vi "AutoRun.vi"(11 "AllControls In":T1) -> ()   [LabVIEW 2017]
uses:
  Ctrls/AllControls.ctl
  Ctrls/Data.ctl
  Ctrls/CSV_Data.ctl
  <vilib>/Utility/miscctls.llb/LVRowAndColumnTypeDef.ctl
  Ctrls/AlarmIndex.ctl
  Ctrls/PathChoose.ctl
  <vilib>/Utility/file.llb/Write Delimited Spreadsheet (string).vi
  <vilib>/regexp/Match Regular Expression.xnode
panel:
  out "Station ID":string
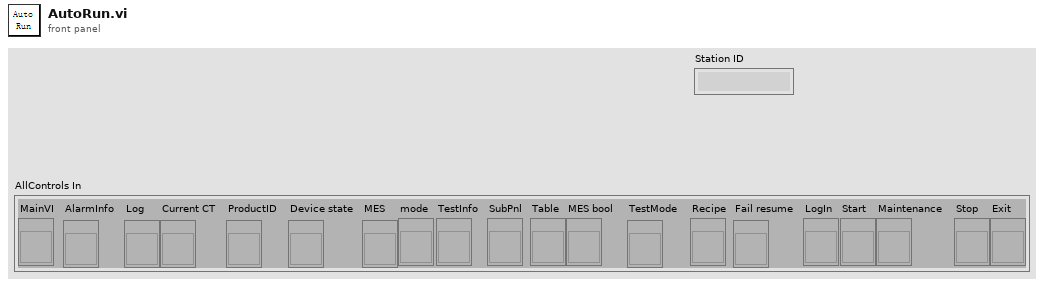
[diagram p1: front panel]
types:
  T1 = typedef "AllControls.ctl" = cluster{"MainVI":refnum<vi>, "AlarmInfo":refnum<vi>, "Log":refnum<vi>, "Current CT":refnum<vi>, "ProductID":refnum<vi>, "Device state":refnum<vi>, "MES":refnum<vi>, "mode":refnum<vi>, "TestInfo":refnum<vi>, "SubPnl":refnum<vi>, "Table":refnum<vi>, "MES bool":refnum<vi>, "TestMode":refnum<vi>, "Recipe":refnum<vi>, "Fail resume":refnum<vi>, "LogIn":refnum<vi>, "Start":refnum<vi>, "Maintenance":refnum<vi>, "Stop":refnum<vi>, "Exit":refnum<vi>}
  T2 = typedef "CSV_Data.ctl" = cluster{"SN":string, "Table":string[][], "Count":cluster{"Total":i32, "OK":i32, "NG":i32, "Yield":dbl}, "Start Time":timestamp, "daemon reference":refnum<k5>, "CT":dbl, "OK/NG":bool, "Station ID":string, "MES DDM SN":string, "MES PCBA SN":string, "Retest":string, "Attachment RFID detection":cluster{"UID":string, "tag content":string}, "SKU":string, "Plate_Diameter":string, "Alarm":string}
  T3 = typedef "Data.ctl" = cluster{"Initialisation":cluster{"DDM_Parameter":dbl[], "DDM_Parameter_status":bool[], "Get_Tester_Parameter":dbl[], "Get_Tester_Parameter_status":bool[], "Cal_Tester_Parameter":dbl[], "Cal_Tester_Parameter_status":bool[], "sw_version_before_status":bool, "sw_version_after_status":bool, "Set_SKU_Config_With_LMT_status":bool, "FCT_timestamp_status":bool, "LMT_Connect_to_UUT_status":bool}, "BEMF_Calibration":cluster{"Read_ambient_temperature":dbl, "Calibration_Vaule":dbl[], "Calibration_Vaule _B":dbl[], "Calibration_Vaule_status":bool[], "Calibration_Vaule_B_status":bool[]}, "ECO":cluster{"DDM_Parameter":dbl[], "DDM_Parameter_status":bool[], "Get_Tester_Parameter":dbl[], "Get_Tester_Parameter_status":bool[], "Cal_Tester_Parameter":dbl[], "Cal_Tester_Parameter_status":bool[], "DDM_Parameter_after_power_tune":dbl[], "Get_Tester_Parameter_after_power_tune":dbl[], "Cal_Tester_Parameter_after_power_tune":dbl[], "Cal_Tester_Parameter_after_power_tune_status":bool[], "Delta_P":dbl}, "BOOST":cluster{"DDM_Parameter":dbl[], "DDM_Parameter_status":bool[], "Get_Tester_Parameter":dbl[], "Get_Tester_Parameter_status":bool[], "Cal_Tester_Parameter":dbl[], "Cal_Tester_Parameter_status":bool[], "DDM_Parameter_after_power_tune":dbl[], "Get_Tester_Parameter_after_power_tune":dbl[], "Cal_Tester_Parameter_after_power_tune":dbl[], "Cal_Tester_Parameter_after_power_tune_status":bool[], "airwatts_am_off":dbl, "AW_Delta_(AM_on_and_off)":dbl, "AW_Delta_(AM_on_and_off)_Status":bool, "Delta_P":dbl}, "MAX":cluster{"Average_Tmag_Data":cluster{"LSI Delta in degC":dbl, "FISF Delta in degc":dbl, "LSI Tmag in degC":dbl, "Fisf Tmag in degC":dbl, "IIR Tmag in degC":dbl}, "DDM_Parameter":dbl[], "DDM_Parameter_status":bool[], "Get_Tester_Parameter":dbl[], "Get_Tester_Parameter_status":bool[], "Cal_Tester_Parameter":dbl[], "BEMF_Finetune":cluster{"eol_bemf_mp_cold_coef_c":dbl, "eol_cold_bemf_fisf_offset":dbl}, "AW_Tune":cluster{"delta_P1":dbl, "delta_P_Setting":dbl}, "DDM_Parameter_after_Airwatts_Tune":dbl[], "Get_Tester_Parameter_after_Airwatts_Tune":dbl[], "Cal_Tester_Parameter_after_Airwatts_Tune":dbl[], "DDM_Parameter_after_Airwatts_Finetune":dbl[], "Get_Tester_Parameter_after_Airwatts_Finetune":dbl[], "Cal_Tester_Parameter_after_Airwatts_Finetune":dbl[], "AW_Finetune":cluster{"delta_P2":dbl, "delta_P_Setting":dbl}, "Delta_Tmag_after_tune":cluster{"LSI Delta in degC":dbl, "FISF Delta in degc":dbl, "LSI Tmag in degC":dbl, "Fisf Tmag in degC":dbl, "IIR Tmag in degC":dbl}, "Hot Bemf in mV":dbl, "DDM_Pressure":dbl, "Delta_Pressure":dbl, " Cold Bemf in mV":dbl, " delta Bemf":dbl, " delta p":dbl, "Delta_Pressure_status":bool, " delta Bemf_status":bool, "LSI Delta in degC_status":bool, "FISF Delta in degc_status":bool, "Max_check_derate_status_status":bool, "Average_All_data":dbl[][], "Average_Tmag_Data_status":bool[], "Average_Tmag_Data_after_tune_status":bool[], "Cal_Tester_Parameter_status":bool[], "Cal_Tester_Parameter_status_after_Airwatts_Tune":bool[], "Cal_Tester_Parameter_status_after_Airwatts_FineTune":bool[]}, "Task_Detect_Calib":cluster{"LL":cluster{"DDM_Parameter":dbl[], "DDM_Parameter_status":bool[], "Get_Tester_Parameter":dbl[], "Get_Tester_Parameter_status":bool[], "Set_task_detect_A":dbl, "Set_task_detect_A_Status":bool}, "HL":cluster{"DDM_Parameter":dbl[], "DDM_Parameter_status":bool[], "Get_Tester_Parameter":dbl[], "Get_Tester_Parameter_status":bool[], "Set_task_detect_B":dbl, "Set_task_detect_B_Status":bool}, "LH":cluster{"DDM_Parameter":dbl[], "DDM_Parameter_status":bool[], "Get_Tester_Parameter":dbl[], "Get_Tester_Parameter_status":bool[], "Set_task_detect_C":dbl, "Set_task_detect_C_Status":bool}, "HH":cluster{"DDM_Parameter":dbl[], "DDM_Parameter_status":bool[], "Get_Tester_Parameter":dbl[], "Get_Tester_Parameter_status":bool[], "Set_task_detect_D":dbl, "Read_and_check_calibration_Status":bool[], "Set_task_detect_D_Status":bool}, "Get_eol_inlet_blockage_E":dbl, "Calib_vaule":cluster{"Get_task_detect_LL":dbl, "Get_task_detect_HL":dbl, "Get_task_detect_LH":dbl, "Get_task_detect_HH":dbl, "eol_inlet_blockage":dbl, "eol_code_bemf_temp":dbl}, "calibrated temp":dbl, "Inlet_Blockage_Calibration":cluster{"DDM_Parameter":dbl[], "DDM_Parameter_status":bool[], "Get_Tester_Parameter":dbl[], "Get_Tester_Parameter_status":bool[]}, "Get_eol_inlet_blockage_E_Status":bool}, "good":cluster{"Write_Product_TS":cluster{"TIMESTAMP":i64, "RIG_ID":i64, "PASSMARK_ID":i64, "PASSMARK_REV":i64}, "Read_Product_TS":cluster{"TIMESTAMP":i64, "RIG_ID":i64, "PASSMARK_ID":i64, "PASSMARK_REV":i64}, "Good_Check_Secuity_Bit_Stauts":bool}}
  T4 = typedef "HD Config.ctl" = cluster{" PC":cluster{"PC Address":u8[], "PC Port":i32}, "FCO":cluster{"COM":refnum<visa-resource-name>, "Baudrate":u32}, "DC Power ":cluster{"COM":refnum<visa-resource-name>, "Baudrate":u32}, "PW3336":cluster{"COM":refnum<visa-resource-name>, "Baudrate":u32}, "Lefoo":cluster{"COM":refnum<visa-resource-name>, "Baudrate":u32}, "AI Model":cluster{"COM":refnum<visa-resource-name>, "Baudrate":u32}, "DIPC":cluster{"COM":refnum<visa-resource-name>}, "RFID":cluster{"IP Address":string, "Port":u16, "Retry":u16}, "Motor":cluster{"COM":refnum<visa-resource-name>, "Baudrate":u32}, "Fail_resume_mode":bool, "GRR":bool}
  T5 = typedef "amc_Message Queue.ctl" = refnum<queue>
  T6 = typedef "TesterInfo.ctl" = cluster{"Station Name":string, "Station Code":string, "ES NO.":string, "Tester ID":string, "PassMark Revision":string, "Rig ID":string, "Deamon_vision":string, "Project Name":string, "FFTesterPath":path, "Enable_User":bool, "Mode":enum16{"682"}, "MES":bool}
  T7 = cluster{"Total":i32, "OK":i32, "NG":i32, "Yield":dbl}
  T8 = typedef "LVRowAndColumnTypeDef.ctl" = cluster{"Row":i32, "Column":i32}
  T9 = enum8{"Enabled", "Disabled", "Disabled and Grayed Out"}
  T10 = typedef "AlarmIndex.ctl" = enum16{"E-Stop", "Safety light grid", "UUT Sealing Cylinder HomePoint", "UUT Sealing Cylinder WorkPoint", "Orifice fixed Cylinder L HomePoint", "Orifice fixed Cylinder L WorkPoint", "Orifice fixed Cylinder R HomePoint", "Orifice fixed Cylinder R WorkPoint", "UUT Cylinder HomePoint", "UUT Cylinder WorkPoint", "Carrier fixed Cylinder L HomePoint", "Carrier fixed Cylinder L WorkPoint", "Carrier fixed Cylinder R HomePoint", "Carrier fixed Cylinder R WorkPoint", "Probe Cylinder HomePoint", "Probe Cylinder WorkPoint", "Motor Error", "Test Error"}
  T11 = typedef "PathChoose.ctl" = enum16{"OperatorLog", "AutoRunLog", "AlmLog", "TestData", "AllTestData", "backup_nvm", "backup_before_flashing"}
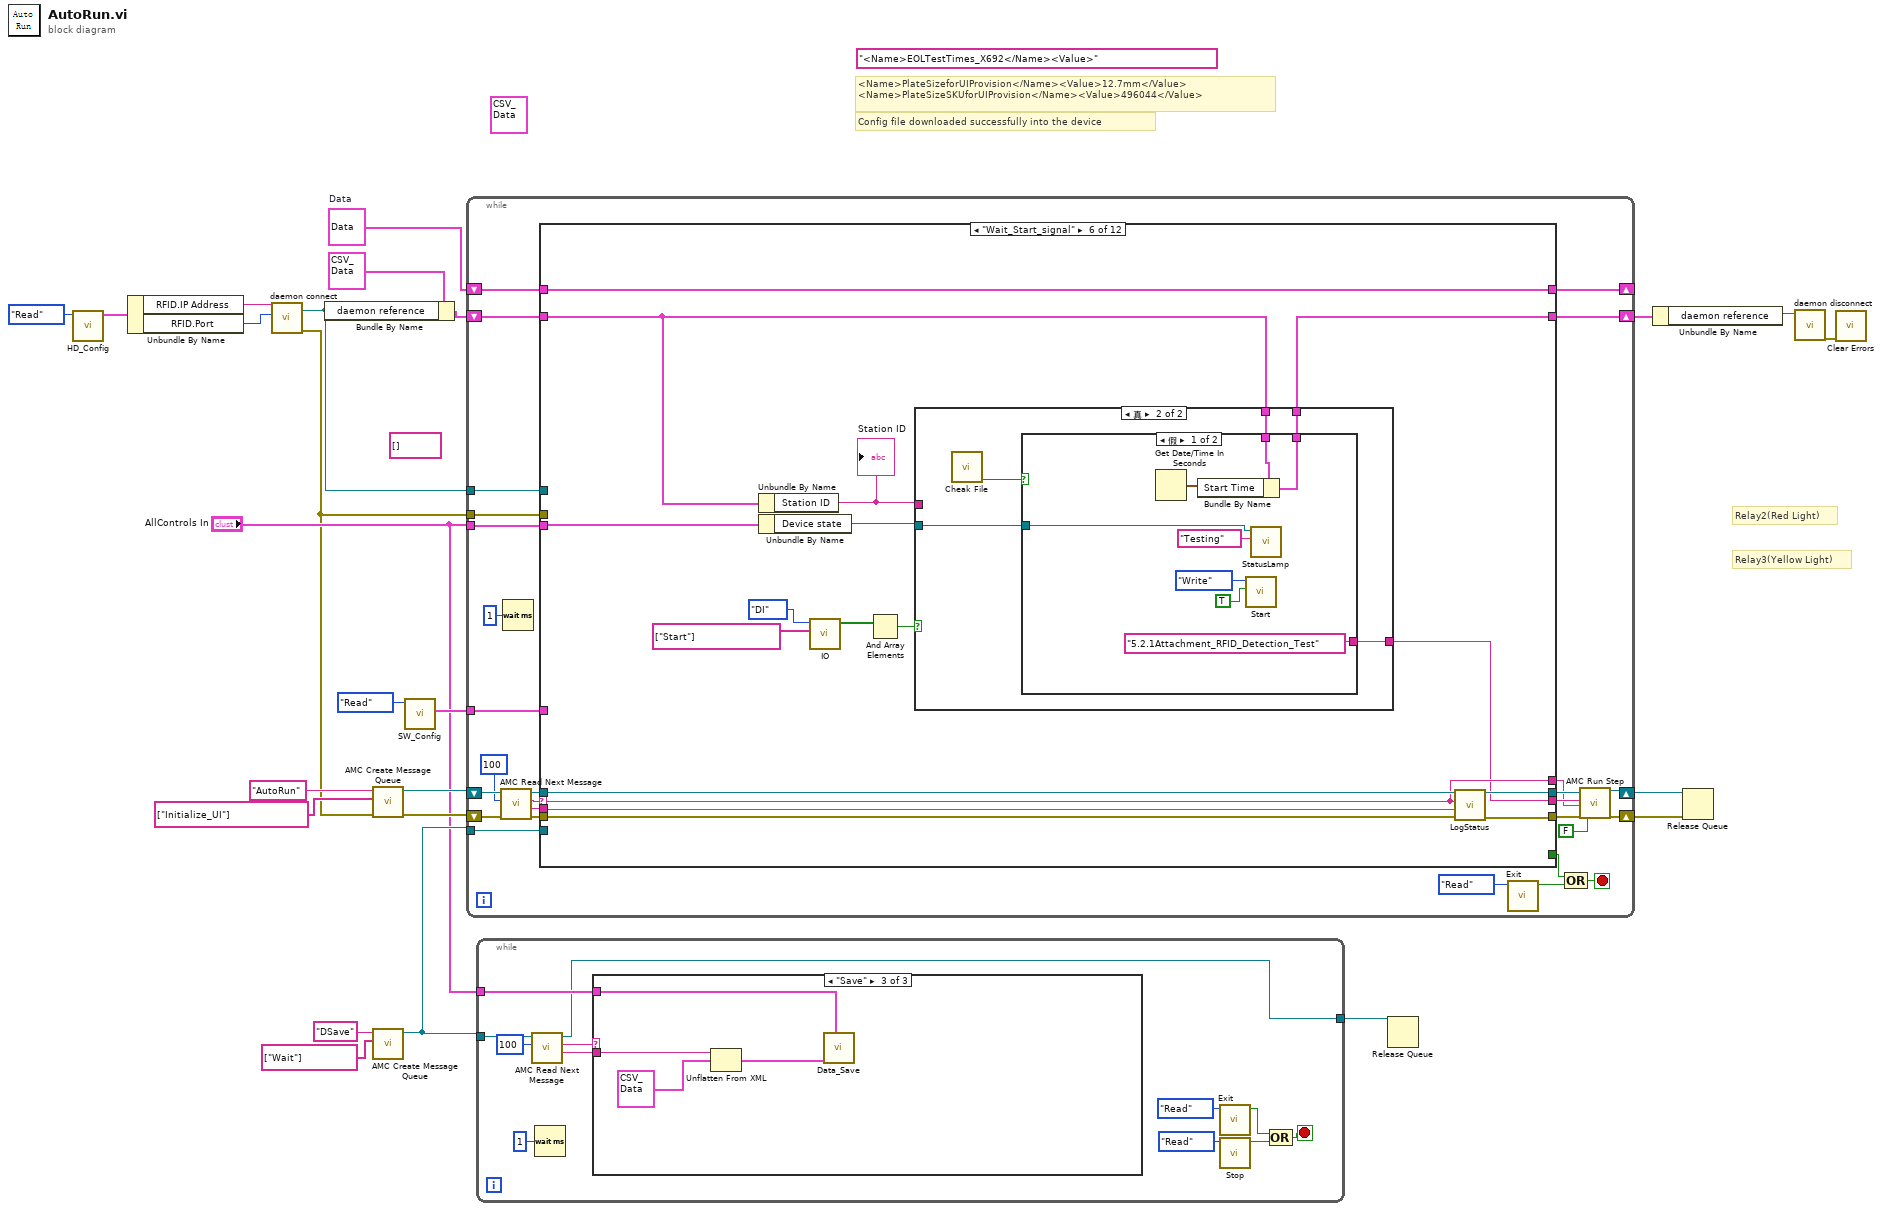
[diagram p0: block diagram]
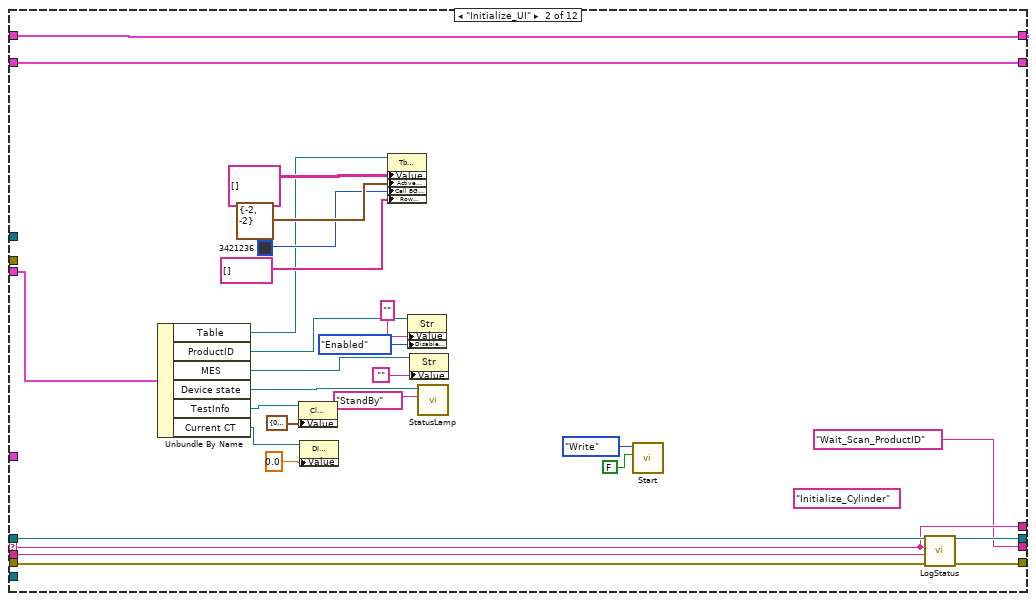
[diagram p5: hidden frame]
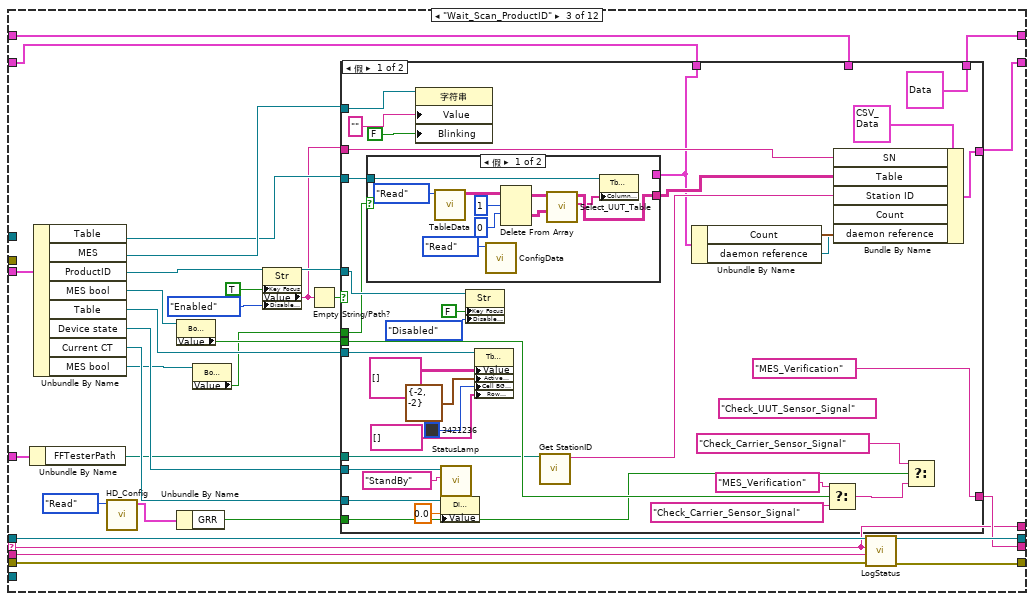
[diagram p6: hidden frame]
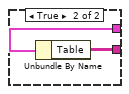
[diagram p7: hidden frame]
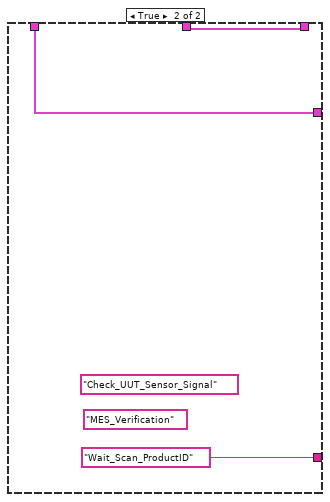
[diagram p8: hidden frame]
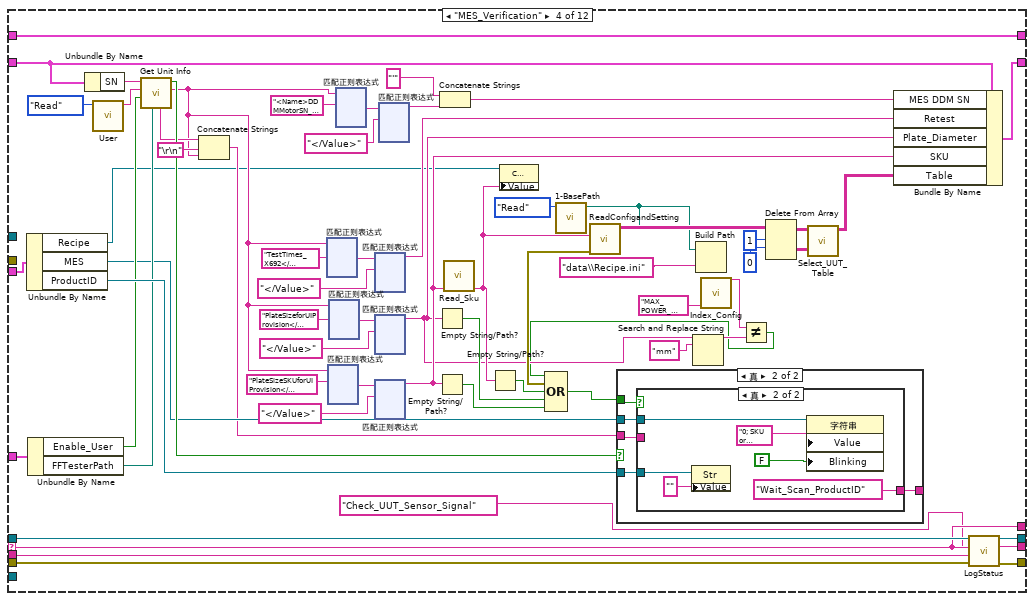
[diagram p9: hidden frame]
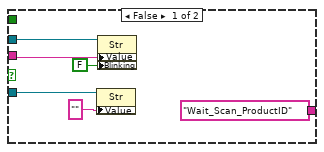
[diagram p10: hidden frame]
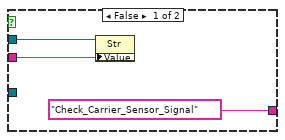
[diagram p11: hidden frame]
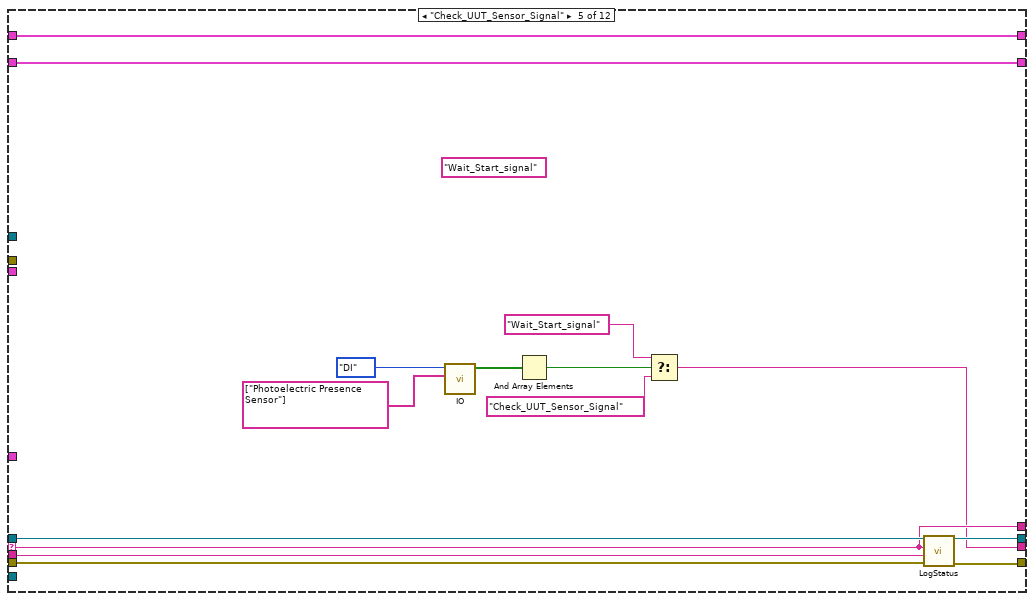
[diagram p12: hidden frame]
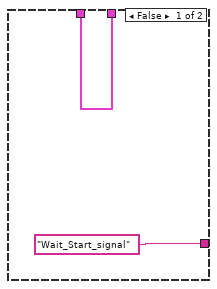
[diagram p13: hidden frame]
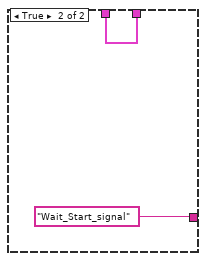
[diagram p14: hidden frame]
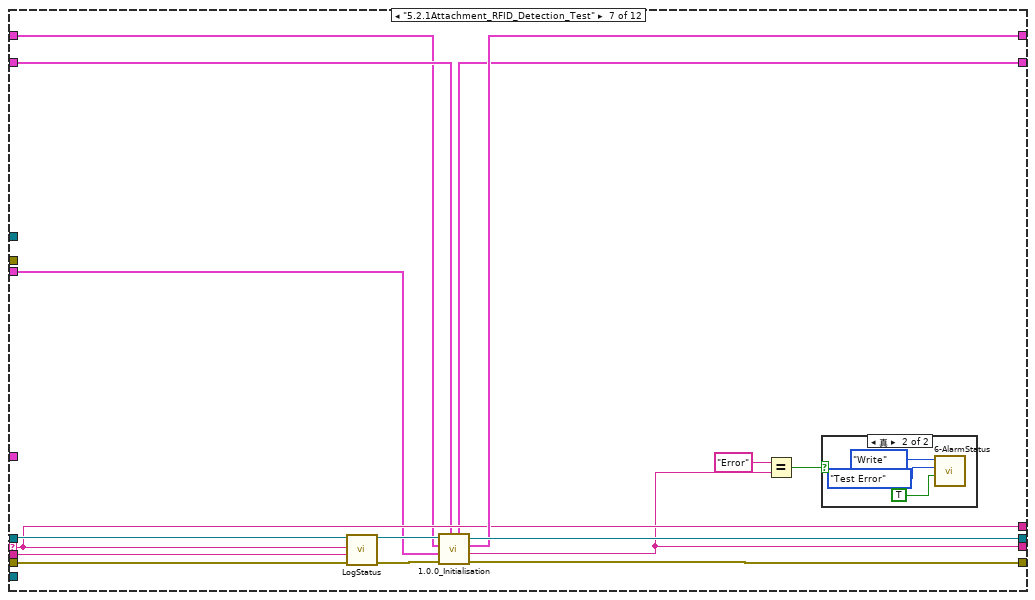
[diagram p15: hidden frame]
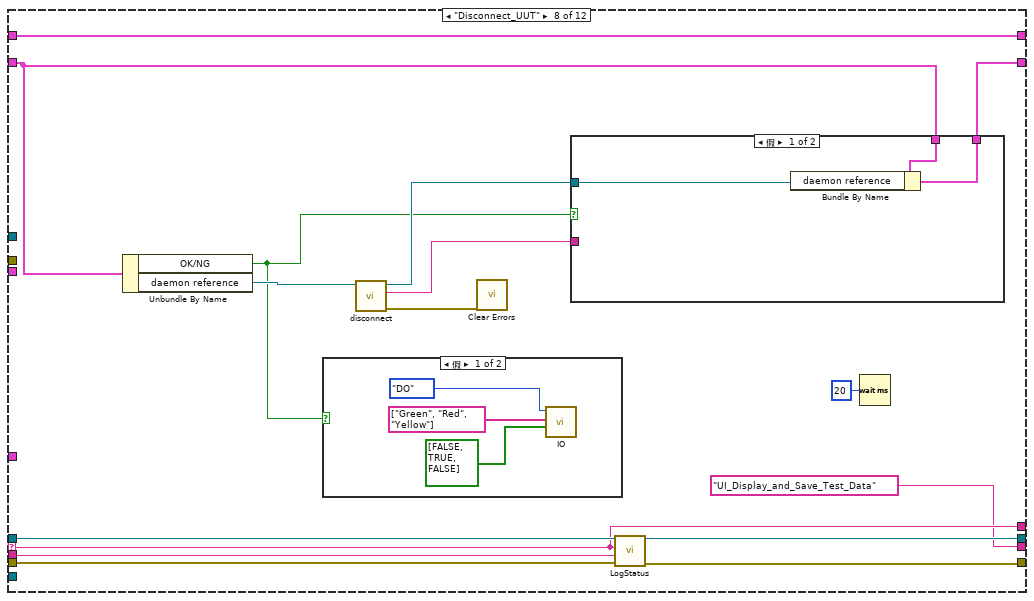
[diagram p17: hidden frame]
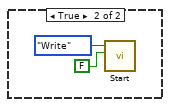
[diagram p18: hidden frame]
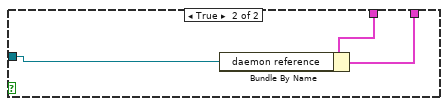
[diagram p19: hidden frame]
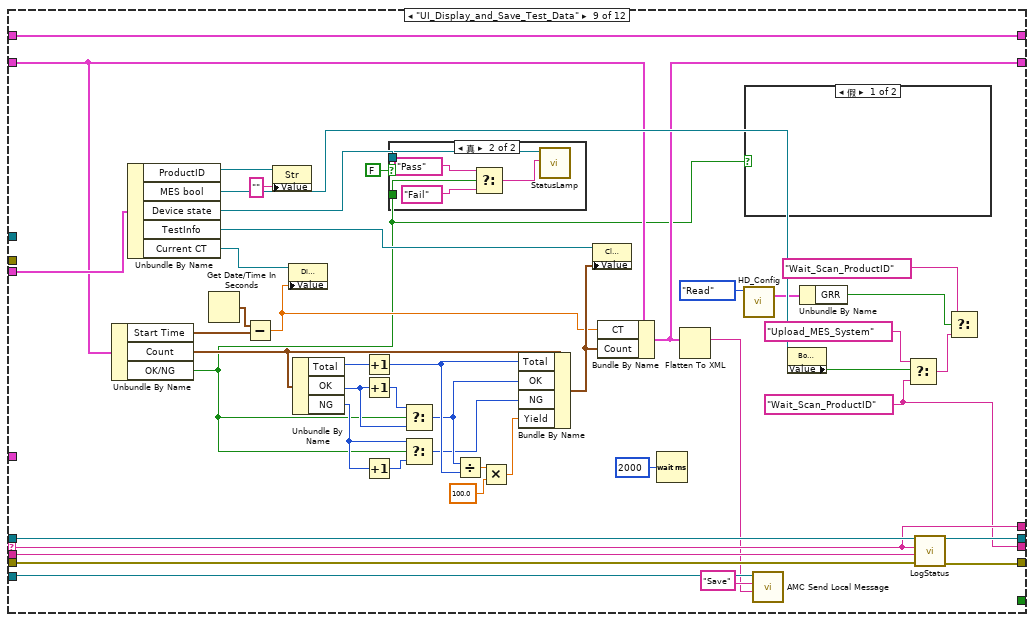
[diagram p20: hidden frame]
diagram:
  (unwired) T2 {"SN"="", "Table"=[], "Count"={"Total"=0, "OK"=0, "NG"=0, "Yield"=0.0}, "Start Time"=timestamp(0 s since 1904-01-01), "daemon reference"=refnum, "CT"=0.0, "OK/NG"=FALSE, "Station ID"="", "MES DDM SN"="", "MES PCBA SN"="", "Retest"="", "Attachment RFID detection"={"UID"="", "tag content"=""}, "SKU"="", "Plate_Diameter"="", "Alarm"=""} ("Data in")
  (unwired) string[] []
  (unwired) "<Name>EOLTestTimes_X692</Name><Value>" ("正则表达式")
  w8 = T3 {"Initialisation"={"DDM_Parameter"=[], "DDM_Parameter_status"=[], "Get_Tester_Parameter"=[], "Get_Tester_Parameter_status"=[], "Cal_Tester_Parameter"=[], "Cal_Tester_Parameter_status"=[], "sw_version_before_status"=FALSE, "sw_version_after_status"=FALSE, "Set_SKU_Config_With_LMT_status"=FALSE, "FCT_timestamp_status"=FALSE, "LMT_Connect_to_UUT_status"=FALSE}, "BEMF_Calibration"={"Read_ambient_temperature"=0.0, "Calibration_Vaule"=[], "Calibration_Vaule _B"=[], "Calibration_Vaule_status"=[], "Calibration_Vaule_B_status"=[]}, "ECO"={"DDM_Parameter"=[], "DDM_Parameter_status"=[], "Get_Tester_Parameter"=[], "Get_Tester_Parameter_status"=[], "Cal_Tester_Parameter"=[], "Cal_Tester_Parameter_status"=[], "DDM_Parameter_after_power_tune"=[], "Get_Tester_Parameter_after_power_tune"=[], "Cal_Tester_Parameter_after_power_tune"=[], "Cal_Tester_Parameter_after_power_tune_status"=[], "Delta_P"=0.0}, "BOOST"={"DDM_Parameter"=[], "DDM_Parameter_status"=[], "Get_Tester_Parameter"=[], "Get_Tester_Parameter_status"=[], "Cal_Tester_Parameter"=[], "Cal_Tester_Parameter_status"=[], "DDM_Parameter_after_power_tune"=[], "Get_Tester_Parameter_after_power_tune"=[], "Cal_Tester_Parameter_after_power_tune"=[], "Cal_Tester_Parameter_after_power_tune_status"=[], "airwatts_am_off"=0.0, "AW_Delta_(AM_on_and_off)"=0.0, "AW_Delta_(AM_on_and_off)_Status"=FALSE, "Delta_P"=0.0}, "MAX"={"Average_Tmag_Data"={"LSI Delta in degC"=0.0, "FISF Delta in degc"=0.0, "LSI Tmag in degC"=0.0, "Fisf Tmag in degC"=0.0, "IIR Tmag in degC"=0.0}, "DDM_Parameter"=[], "DDM_Parameter_status"=[], "Get_Tester_Parameter"=[], "Get_Tester_Parameter_status"=[], "Cal_Tester_Parameter"=[], "BEMF_Finetune"={"eol_bemf_mp_cold_coef_c"=0.0, "eol_cold_bemf_fisf_offset"=0.0}, "AW_Tune"={"delta_P1"=0.0, "delta_P_Setting"=0.0}, "DDM_Parameter_after_Airwatts_Tune"=[], "Get_Tester_Parameter_after_Airwatts_Tune"=[], "Cal_Tester_Parameter_after_Airwatts_Tune"=[], "DDM_Parameter_after_Airwatts_Finetune"=[], "Get_Tester_Parameter_after_Airwatts_Finetune"=[], "Cal_Tester_Parameter_after_Airwatts_Finetune"=[], "AW_Finetune"={"delta_P2"=0.0, "delta_P_Setting"=0.0}, "Delta_Tmag_after_tune"={"LSI Delta in degC"=0.0, "FISF Delta in degc"=0.0, "LSI Tmag in degC"=0.0, "Fisf Tmag in degC"=0.0, "IIR Tmag in degC"=0.0}, "Hot Bemf in mV"=0.0, "DDM_Pressure"=0.0, "Delta_Pressure"=0.0, " Cold Bemf in mV"=0.0, " delta Bemf"=0.0, " delta p"=0.0, "Delta_Pressure_status"=FALSE, " delta Bemf_status"=FALSE, "LSI Delta in degC_status"=FALSE, "FISF Delta in degc_status"=FALSE, "Max_check_derate_status_status"=FALSE, "Average_All_data"=[], "Average_Tmag_Data_status"=[], "Average_Tmag_Data_after_tune_status"=[], "Cal_Tester_Parameter_status"=[], "Cal_Tester_Parameter_status_after_Airwatts_Tune"=[], "Cal_Tester_Parameter_status_after_Airwatts_FineTune"=[]}, "Task_Detect_Calib"={"LL"={"DDM_Parameter"=[], "DDM_Parameter_status"=[], "Get_Tester_Parameter"=[], "Get_Tester_Parameter_status"=[], "Set_task_detect_A"=0.0, "Set_task_detect_A_Status"=FALSE}, "HL"={"DDM_Parameter"=[], "DDM_Parameter_status"=[], "Get_Tester_Parameter"=[], "Get_Tester_Parameter_status"=[], "Set_task_detect_B"=0.0, "Set_task_detect_B_Status"=FALSE}, "LH"={"DDM_Parameter"=[], "DDM_Parameter_status"=[], "Get_Tester_Parameter"=[], "Get_Tester_Parameter_status"=[], "Set_task_detect_C"=0.0, "Set_task_detect_C_Status"=FALSE}, "HH"={"DDM_Parameter"=[], "DDM_Parameter_status"=[], "Get_Tester_Parameter"=[], "Get_Tester_Parameter_status"=[], "Set_task_detect_D"=0.0, "Read_and_check_calibration_Status"=[], "Set_task_detect_D_Status"=FALSE}, "Get_eol_inlet_blockage_E"=0.0, "Calib_vaule"={"Get_task_detect_LL"=0.0, "Get_task_detect_HL"=0.0, "Get_task_detect_LH"=0.0, "Get_task_detect_HH"=0.0, "eol_inlet_blockage"=0.0, "eol_code_bemf_temp"=0.0}, "calibrated temp"=0.0, "Inlet_Blockage_Calibration"={"DDM_Parameter"=[], "DDM_Parameter_status"=[], "Get_Tester_Parameter"=[], "Get_Tester_Parameter_status"=[]}, "Get_eol_inlet_blockage_E_Status"=FALSE}, "good"={"Write_Product_TS"={"TIMESTAMP"=0, "RIG_ID"=0, "PASSMARK_ID"=0, "PASSMARK_REV"=0}, "Read_Product_TS"={"TIMESTAMP"=0, "RIG_ID"=0, "PASSMARK_ID"=0, "PASSMARK_REV"=0}, "Good_Check_Secuity_Bit_Stauts"=FALSE}}  # Data
  # "Relay3(Yellow Light)"
  # "Relay2(Red Light)"
  # "<Name>PlateSizeforUIProvision</Name><Value>12.7mm</Value>\n<Name>PlateSizeSKUforUIProvision</Name><Value>496044</Value>"
  # "Config file downloaded successfully into the device"
  n1 = call "HD_Config.vi"("Step"=enum16{"Initial", "Write", "Read"}."Read") -> ("HD Config out"=w16:T4)  [unwired: 9 in, 1 out]
  n2 = Unbundle By Name(w16) -> ("RFID.IP Address"=w14:string, "RFID.Port"=w13:u16)
  n3 = call "daemon connect.vi"("port (6543)"=w13, "address (localhost)"=w14) -> ("error out"=w2:errorcluster, "daemon reference out"=w3:refnum<k5>)  [unwired: 8 in]
  n4 = Bundle By Name(cluster=T2 {"SN"="", "Table"=[], "Count"={"Total"=0, "OK"=0, "NG"=0, "Yield"=0.0}, "Start Time"=timestamp(0 s since 1904-01-01), "daemon reference"=refnum, "CT"=0.0, "OK/NG"=FALSE, "Station ID"="", "MES DDM SN"="", "MES PCBA SN"="", "Retest"="", "Attachment RFID detection"={"UID"="", "tag content"=""}, "SKU"="", "Plate_Diameter"="", "Alarm"=""} ("Data in"), "daemon reference"=w3) -> (w10:T2)
  n5 = call "AMC Create Message Queue.vi"("error in (no error)"=w2, "Initial Message Names"=string[] ["Initialize_UI"] ("Initial Message Values"), "Message Queue Name"="AutoRun" ("Message queue name (unnamed)")) -> ("error out"=w23:errorcluster, "Message Queue out"=w24:T5)  [unwired: 2 in, 5 out]
  n6 = call "AMC Create Message Queue.vi"("Initial Message Names"=string[] ["Wait"], "Message Queue Name"="DSave") -> ("Message Queue out"=w19:T5)  [unwired: 3 in, 6 out]
  n7 = call "SW_Config.vi"("Step"=enum16{"Initial", "Write", "Read"}."Read") -> ("SW Config out"=w11:T6)  [unwired: 9 in, 1 out]
  n8 = while {
    tunnel: "AllControls In" -> [w39]
    shift-right: [w48] -> w6
    shift-left: w24 -> [w53]
    shift-right: [w49] -> w5
    shift-left: w23 -> [w52]
    tunnel: w19 -> [w44]
    shift-right: [w31] -> _
    shift-left: w8 -> [w32]
    tunnel: w11 -> [w30]
    shift-right: [w29] -> w9
    shift-left: w10 -> [w28]
    tunnel: w3 -> [w27]
    tunnel: w2 -> [w26]
    stop <- w47 stop-if-true
    n9 = call "AMC Read Next Message.vi"("error in (no error)"=w52, "timeout (1ms)"=100 ("Timeout"), "Message Queue in"=w53) -> ("error out"=w40:errorcluster, "Message Value"=w33:string, "Message Name"=w43:string, "Message Queue out"=w42:T5)  [unwired: 1 in, 4 out]
    n10 = Wait (ms)(milliseconds to wait=u32 1) -> ()  [unwired: 1 out]
    n11 = case shown="\"Wait_Start_signal\"" w43 {
      selector: w43 -> [_ w73 w102 w220 w1165 w1183 w1214 w1235 w1289 w1319 w1361 w1374]
      tunnel: w44 -> [_ _ _ _ _ _ _ _ w1293 _ _ _]
      tunnel: w42 -> [w57 w84 w115 w226 w1172 w1188 w1218 w1238 w1294 w1324 w1364 w1376]
      tunnel: [w57 w84 w115 w226 w1172 w1188 w1217 w1238 w1294 w1324 w1364 w1376] -> w41
      tunnel: w40 -> [w56 w63 w114 w225 w1171 w1187 w1220 w1237 w1291 w1323 w1363 w1371]
      tunnel: [w56 w80 w113 w224 w1170 w1186 w1216 w1236 w1290 w1322 w1362 w1373] -> w36
      tunnel: w39 -> [_ w82 w109 w222 _ w1180 w1210 _ w1280 w1303 w1352 _]
      tunnel: [_ _ _ _ _ _ _ _ _ _ _ TRUE] -> w38
      tunnel: [_ "Wait_Scan_ProductID" w107 "Check_UUT_Sensor_Signal" ("Name") w1159 w1178 w1207 "UI_Display_and_Save_Test_Data" ("Name") w1253 "Wait_Scan_ProductID" w1353 _] -> w35
      tunnel: [_ w73 w102 w220 w1165 w1183 w1214 w1235 w1289 w1319 w1361 _] -> w34
      tunnel: w33 -> [_ w74 w105 w221 w1164 w1182 w1219 w1234 w1288 w1320 w1360 _]
      tunnel: w32 -> [w55 w60 w103 w212 w1166 w1175 w1206 w1229 w1261 w1318 w1346 w1372]
      tunnel: [w55 w60 w104 w212 w1166 w1175 w1215 w1229 w1261 w1318 w1346 w1372] -> w31
      tunnel: w30 -> [_ _ w95 w215 _ _ _ _ _ w1305 _ _]
      tunnel: [w54 w59 w93 w210 w1160 w1174 w1209 w1230 w1260 w1302 w1336 w1370] -> w29
      tunnel: w28 -> [w54 w59 w92 w211 w1160 w1176 w1208 w1228 w1259 w1302 w1336 w1370]
      tunnel: w27 -> [_ _ _ _ _ _ _ _ _ _ _ w1369]
      tunnel: w26 -> [_ _ _ _ _ _ _ _ _ _ _ w1368]
      frame "Empty", Default {
      }
      frame "Initialize_UI" {
        (unwired) "Initialize_Cylinder"
        n12 = Unbundle By Name(w82) -> ("Table"=w68:refnum<vi>, "ProductID"=w77:refnum<vi>, "MES"=w83:refnum<vi>, "Device state"=w79:refnum<vi>, "TestInfo"=w67:refnum<vi>, "Current CT"=w65:refnum<vi>)
        n13 = property class="Clust (strict)"(reference=w67, "Value"=T7 {"Total"=0, "OK"=0, "NG"=0, "Yield"=0.0}) -> ()  [unwired: 1 in, 2 out]
        n14 = property class="DigNum (strict)"(reference=w65, "Value"=0.0) -> ()  [unwired: 1 in, 2 out]
        n15 = property class="Tbl (strict)"(reference=w68, "Value"=string[][] [] ("值"), "Active Cell"=T8 {"Row"=-2, "Column"=-2} ("活动单元格:活动单元格"), "Cell BG Color"=u32 3421236, "Row Headers[]"=string[] [] ("Row Header Strings[]")) -> ()  [unwired: 1 in, 2 out]
        n16 = property class="Str"(reference=w77, "Value"="" ("值"), "DisabledEnum"=T9."Enabled" ("Disabled")) -> ()  [unwired: 1 in, 2 out]
        n17 = property class="Str"(reference=w83, "Value"="") -> ()  [unwired: 1 in, 2 out]
        n18 = call "StatusLamp.vi"("State"="StandBy", "Boolean输入"=w79) -> ()  [unwired: 9 in, 1 out]
        n19 = call "Start.vi"("Start In"=FALSE, "Step"=enum16{"Initial", "Write", "Read"}."Write") -> ()  [unwired: 8 in, 2 out]
        n20 = call "LogStatus.vi"("error in (no error)"=w63, "last message"=w74, "message"=w73) -> ("error  out"=w80:errorcluster)  [unwired: 8 in]
      }
      frame "Wait_Scan_ProductID" {
        n21 = Unbundle By Name(w95) -> ("FFTesterPath"=w94:path)
        n22 = Unbundle By Name(w109) -> ("Table"=w86:refnum<vi>, "MES"=w99:refnum<vi>, "ProductID"=w112:refnum<vi>, "MES bool"=w101:refnum<vi>, "Table"=w98:refnum<vi>, "Device state"=w97:refnum<vi>, "Current CT"=w96:refnum<vi>, "MES bool"=w88:refnum<vi>)
        n23 = call "HD_Config.vi"("Step"=enum16{"Initial", "Write", "Read"}."Read") -> ("HD Config out"=w90:T4)  [unwired: 9 in, 1 out]
        n24 = property class="Bool (strict)"(reference=w101) -> ("Value"=w100:bool)  [unwired: 1 in, 2 out]
        n25 = Unbundle By Name(w90) -> ("GRR"=w89:bool)
        n26 = property class="Bool (严格)"(reference=w88) -> ("Value"=w87:bool)  [unwired: 1 in, 2 out]
        n27 = property class="Str"(reference=w112, "Key Focus"=TRUE, "DisabledEnum"=T9."Enabled" ("Disabled")) -> (reference out=w106:refnum<vi>, "Value"=w85:string)  [unwired: 1 in, 1 out]
        n28 = Empty String/Path?(string/path=w85) -> (empty?=w108:bool)
        n29 = case shown="假" w108 {
          tunnel: ["MES_Verification" "Wait_Scan_ProductID"] -> w107
          tunnel: w106 -> [w147 _]
          tunnel: w103 -> [_ w164]
          tunnel: w85 -> [w130 _]
          tunnel: [T3 {"Initialisation"={"DDM_Parameter"=[nan, nan, nan, nan, nan], "DDM_Parameter_status"=[FALSE, FALSE, FALSE, FALSE, FALSE], "Get_Tester_Parameter"=[nan, nan, nan, nan, nan, nan], "Get_Tester_Parameter_status"=[FALSE, FALSE, FALSE, FALSE, FALSE, FALSE], "Cal_Tester_Parameter"=[nan, nan, nan], "Cal_Tester_Parameter_status"=[FALSE, FALSE, FALSE], "sw_version_before_status"=FALSE, "sw_version_after_status"=FALSE, "Set_SKU_Config_With_LMT_status"=FALSE, "FCT_timestamp_status"=FALSE, "LMT_Connect_to_UUT_status"=FALSE}, "BEMF_Calibration"={"Read_ambient_temperature"=nan, "Calibration_Vaule"=[nan, nan, nan, nan, nan, nan, nan, nan, nan, nan], "Calibration_Vaule _B"=[nan, nan], "Calibration_Vaule_status"=[FALSE, FALSE, FALSE, FALSE, FALSE, FALSE, FALSE, FALSE, FALSE, FALSE], "Calibration_Vaule_B_status"=[FALSE, FALSE]}, "ECO"={"DDM_Parameter"=[nan, nan, nan, nan, nan, nan, nan, nan, nan], "DDM_Parameter_status"=[FALSE, FALSE, FALSE, FALSE, FALSE, FALSE, FALSE, FALSE, FALSE], "Get_Tester_Parameter"=[nan, nan, nan, nan, nan, nan, nan], "Get_Tester_Parameter_status"=[FALSE, FALSE, FALSE, FALSE, FALSE, FALSE, FALSE], "Cal_Tester_Parameter"=[nan, nan, nan, nan, nan, nan], "Cal_Tester_Parameter_status"=[FALSE, FALSE, FALSE, FALSE, FALSE], "DDM_Parameter_after_power_tune"=[nan, nan, nan, nan, nan, nan, nan, nan, nan], "Get_Tester_Parameter_after_power_tune"=[nan, nan, nan, nan, nan, nan, nan], "Cal_Tester_Parameter_after_power_tune"=[nan, nan, nan, nan, nan, nan], "Cal_Tester_Parameter_after_power_tune_status"=[FALSE, FALSE, FALSE, FALSE, FALSE], "Delta_P"=nan}, "BOOST"={"DDM_Parameter"=[nan, nan, nan, nan, nan, nan, nan, nan, nan], "DDM_Parameter_status"=[FALSE, FALSE, FALSE, FALSE, FALSE, FALSE, FALSE, FALSE, FALSE], "Get_Tester_Parameter"=[nan, nan, nan, nan, nan, nan, nan], "Get_Tester_Parameter_status"=[FALSE, FALSE, FALSE, FALSE, FALSE, FALSE, FALSE], "Cal_Tester_Parameter"=[nan, nan, nan, nan, nan, nan], "Cal_Tester_Parameter_status"=[FALSE, FALSE, FALSE, FALSE, FALSE], "DDM_Parameter_after_power_tune"=[nan, nan, nan, nan, nan, nan, nan, nan, nan], "Get_Tester_Parameter_after_power_tune"=[nan, nan, nan, nan, nan, nan, nan], "Cal_Tester_Parameter_after_power_tune"=[nan, nan, nan, nan, nan, nan], "Cal_Tester_Parameter_after_power_tune_status"=[FALSE, FALSE, FALSE, FALSE, FALSE], "airwatts_am_off"=nan, "AW_Delta_(AM_on_and_off)"=nan, "AW_Delta_(AM_on_and_off)_Status"=FALSE, "Delta_P"=nan}, "MAX"={"Average_Tmag_Data"={"LSI Delta in degC"=nan, "FISF Delta in degc"=nan, "LSI Tmag in degC"=nan, "Fisf Tmag in degC"=nan, "IIR Tmag in degC"=nan}, "DDM_Parameter"=[nan, nan, nan, nan, nan, nan, nan, nan, nan], "DDM_Parameter_status"=[FALSE, FALSE, FALSE, FALSE, FALSE, FALSE, FALSE, FALSE, FALSE], "Get_Tester_Parameter"=[nan, nan, nan, nan, nan, nan, nan], "Get_Tester_Parameter_status"=[FALSE, FALSE, FALSE, FALSE, FALSE, FALSE, FALSE], "Cal_Tester_Parameter"=[nan, nan, nan, nan, nan, nan], "BEMF_Finetune"={"eol_bemf_mp_cold_coef_c"=nan, "eol_cold_bemf_fisf_offset"=nan}, "AW_Tune"={"delta_P1"=nan, "delta_P_Setting"=nan}, "DDM_Parameter_after_Airwatts_Tune"=[nan, nan, nan, nan, nan, nan, nan, nan, nan], "Get_Tester_Parameter_after_Airwatts_Tune"=[nan, nan, nan, nan, nan, nan, nan], "Cal_Tester_Parameter_after_Airwatts_Tune"=[nan, nan, nan, nan, nan, nan], "DDM_Parameter_after_Airwatts_Finetune"=[nan, nan, nan, nan, nan, nan, nan, nan, nan], "Get_Tester_Parameter_after_Airwatts_Finetune"=[nan, nan, nan, nan, nan, nan, nan], "Cal_Tester_Parameter_after_Airwatts_Finetune"=[nan, nan, nan, nan, nan, nan], "AW_Finetune"={"delta_P2"=nan, "delta_P_Setting"=nan}, "Delta_Tmag_after_tune"={"LSI Delta in degC"=nan, "FISF Delta in degc"=nan, "LSI Tmag in degC"=nan, "Fisf Tmag in degC"=nan, "IIR Tmag in degC"=nan}, "Hot Bemf in mV"=nan, "DDM_Pressure"=nan, "Delta_Pressure"=nan, " Cold Bemf in mV"=nan, " delta Bemf"=nan, " delta p"=nan, "Delta_Pressure_status"=FALSE, " delta Bemf_status"=FALSE, "LSI Delta in degC_status"=FALSE, "FISF Delta in degc_status"=FALSE, "Max_check_derate_status_status"=FALSE, "Average_All_data"=[[nan], [nan], [nan], [nan], [nan]], "Average_Tmag_Data_status"=[FALSE, FALSE, FALSE, FALSE, FALSE], "Average_Tmag_Data_after_tune_status"=[FALSE, FALSE, FALSE, FALSE, FALSE], "Cal_Tester_Parameter_status"=[FALSE, FALSE, FALSE, FALSE, FALSE], "Cal_Tester_Parameter_status_after_Airwatts_Tune"=[FALSE, FALSE, FALSE, FALSE, FALSE], "Cal_Tester_Parameter_status_after_Airwatts_FineTune"=[FALSE, FALSE, FALSE, FALSE, FALSE]}, "Task_Detect_Calib"={"LL"={"DDM_Parameter"=[nan, nan, nan, nan, nan, nan], "DDM_Parameter_status"=[FALSE, FALSE, FALSE, FALSE, FALSE, FALSE], "Get_Tester_Parameter"=[nan, nan, nan, nan], "Get_Tester_Parameter_status"=[FALSE, FALSE, FALSE, FALSE], "Set_task_detect_A"=nan, "Set_task_detect_A_Status"=FALSE}, "HL"={"DDM_Parameter"=[nan, nan, nan, nan, nan, nan], "DDM_Parameter_status"=[FALSE, FALSE, FALSE, FALSE, FALSE, FALSE], "Get_Tester_Parameter"=[nan, nan, nan, nan], "Get_Tester_Parameter_status"=[FALSE, FALSE, FALSE, FALSE], "Set_task_detect_B"=nan, "Set_task_detect_B_Status"=FALSE}, "LH"={"DDM_Parameter"=[nan, nan, nan, nan, nan, nan], "DDM_Parameter_status"=[FALSE, FALSE, FALSE, FALSE, FALSE, FALSE], "Get_Tester_Parameter"=[nan, nan, nan, nan], "Get_Tester_Parameter_status"=[FALSE, FALSE, FALSE, FALSE], "Set_task_detect_C"=nan, "Set_task_detect_C_Status"=FALSE}, "HH"={"DDM_Parameter"=[nan, nan, nan, nan, nan, nan], "DDM_Parameter_status"=[FALSE, FALSE, FALSE, FALSE, FALSE, FALSE], "Get_Tester_Parameter"=[nan, nan, nan, nan], "Get_Tester_Parameter_status"=[FALSE, FALSE, FALSE, FALSE], "Set_task_detect_D"=nan, "Read_and_check_calibration_Status"=[FALSE, FALSE, FALSE, FALSE, FALSE, FALSE], "Set_task_detect_D_Status"=FALSE}, "Get_eol_inlet_blockage_E"=nan, "Calib_vaule"={"Get_task_detect_LL"=nan, "Get_task_detect_HL"=nan, "Get_task_detect_LH"=nan, "Get_task_detect_HH"=nan, "eol_inlet_blockage"=nan, "eol_code_bemf_temp"=nan}, "calibrated temp"=nan, "Inlet_Blockage_Calibration"={"DDM_Parameter"=[nan, nan, nan, nan, nan, nan, nan, nan, nan], "DDM_Parameter_status"=[FALSE, FALSE, FALSE, FALSE, FALSE, FALSE], "Get_Tester_Parameter"=[nan, nan, nan, nan], "Get_Tester_Parameter_status"=[FALSE, FALSE, FALSE, FALSE]}, "Get_eol_inlet_blockage_E_Status"=FALSE}, "good"={"Write_Product_TS"={"TIMESTAMP"=0, "RIG_ID"=0, "PASSMARK_ID"=0, "PASSMARK_REV"=0}, "Read_Product_TS"={"TIMESTAMP"=0, "RIG_ID"=0, "PASSMARK_ID"=0, "PASSMARK_REV"=0}, "Good_Check_Secuity_Bit_Stauts"=FALSE}} ("Data") w164] -> w104
          tunnel: w100 -> [w144 _]
          tunnel: w99 -> [w143 _]
          tunnel: w98 -> [w137 _]
          tunnel: w97 -> [w135 _]
          tunnel: w96 -> [w134 _]
          tunnel: w94 -> [w132 _]
          tunnel: [w131 w163] -> w93
          tunnel: w92 -> [w117 w163]
          tunnel: w89 -> [w126 _]
          tunnel: w87 -> [w119 _]
          tunnel: w86 -> [w118 _]
          frame False {
            (unwired) "Check_UUT_Sensor_Signal" ("Name")
            n30 = case shown="假" w119 {
              tunnel: [w153 w160] -> w129
              tunnel: w118 -> [w151 _]
              tunnel: w117 -> [_ w161]
              frame False {
                n31 = call "TableData.vi"("Step"=enum16{"Initial", "Write", "Read"}."Read") -> ("Tabledata Out"=w154:string[][])  [unwired: 9 in, 1 out]
                n32 = call "ConfigData.vi"("Step"=enum16{"Initial", "Write", "Read"}."Read") -> ()  [unwired: 9 in, 2 out]
                n33 = Delete From Array(array=w154, length=1 ("长度"), index (row)=0 ("索引 (行)")) -> (deleted portion=w155:string[][], array with subset deleted=w156:string[][])  [unwired: 1 in]
                n34 = call "Select_UUT_Table.vi"("all Title"=w155, "all Table"=w156) -> ("Title"=w150:string[], "Table"=w153:string[][])  [unwired: 8 in]
                n35 = property class="Tbl (strict)"(reference=w151, "Column Headers[]"=w150) -> ()  [unwired: 1 in, 2 out]
              }
              frame True {
                n36 = Unbundle By Name(w161) -> ("Table"=w160:string[][])
              }
            }
            n37 = property class="字符串"(reference=w143, "Value"="" ("值"), "Blinking"=FALSE ("闪烁")) -> ()  [unwired: 1 in, 2 out]
            n38 = call "StatusLamp.vi"("State"="StandBy", "Boolean输入"=w135) -> ()  [unwired: 9 in, 1 out]
            n39 = property class="DigNum (strict)"(reference=w134, "Value"=0.0) -> ()  [unwired: 1 in, 2 out]
            n40 = property class="Str"(reference=w147, "Key Focus"=FALSE, "DisabledEnum"=T9."Disabled" ("Disabled")) -> ()  [unwired: 1 in, 2 out]
            n41 = property class="Tbl (strict)"(reference=w137, "Value"=string[][] [] ("值"), "Active Cell"=T8 {"Row"=-2, "Column"=-2} ("活动单元格:活动单元格"), "Cell BG Color"=u32 3421236, "Row Headers[]"=string[] [] ("Row Header Strings[]")) -> ()  [unwired: 1 in, 2 out]
            n42 = call "Get StationID.vi"("路径"=w132) -> ("Station ID"=w128:string)  [unwired: 10 in]
            n43 = Unbundle By Name(w117) -> ("Count"=w123:T7, "daemon reference"=w122:refnum<k5>)
            n44 = Select(t="MES_Verification", s=w144, f="Check_Carrier_Sensor_Signal") -> (s? t:f=w127:string)
            n45 = Bundle By Name(cluster=T2 {"SN"="", "Table"=[], "Count"={"Total"=0, "OK"=0, "NG"=0, "Yield"=0.0}, "Start Time"=timestamp(0 s since 1904-01-01), "daemon reference"=refnum, "CT"=0.0, "OK/NG"=FALSE, "Station ID"="", "MES DDM SN"="", "MES PCBA SN"="", "Retest"="", "Attachment RFID detection"={"UID"="", "tag content"=""}, "SKU"="", "Plate_Diameter"="", "Alarm"=""} ("Data in"), "SN"=w130, "Table"=w129, "Station ID"=w128, "Count"=w123, "daemon reference"=w122) -> (w131:T2)
            n46 = Select(t="Check_Carrier_Sensor_Signal", s=w126, f=w127) -> ()  [unwired: 1 out]
          }
          frame True {
            (unwired) "Check_UUT_Sensor_Signal" ("Name")
            (unwired) "MES_Verification"
          }
        }
        n47 = call "LogStatus.vi"("error in (no error)"=w114, "last message"=w105, "message"=w102) -> ("error  out"=w113:errorcluster)  [unwired: 8 in]
      }
      frame "MES_Verification" {
        n48 = Unbundle By Name(w222) -> ("Recipe"=w165:refnum<vi>, "MES"=w197:refnum<vi>, "ProductID"=w218:refnum<vi>)
        n49 = Unbundle By Name(w215) -> ("Enable_User"=w214:bool, "FFTesterPath"=w213:path)
        n50 = Unbundle By Name(w211) -> ("SN"=w223:string)
        n51 = call "User.vi"("Step"=enum16{"Initial", "Write", "Read"}."Read") -> ("User out"=w216:string)  [unwired: 9 in, 1 out]
        n52 = call "Get Unit Info.vi"("路径"=w213, "Enable_User"=w214, "UserID"=w216, "Serial Number"=w223) -> ("strUnitInfo"=w189:string, "Operation Success"=w219:bool, "结果字符串"=w203:string)  [unwired: 2 in, 3 out]
        n53 = Concatenate Strings(w203, "\r\n", w189) -> (w196:string)
        n54 = xnode "匹配正则表达式"("输入字符串"=w189, "正则表达式"="TestTimes_X692</Name><Value>") -> ("匹配之后"=w201:string)  [unwired: 4 in, 4 out]
        n55 = xnode "匹配正则表达式"("输入字符串"=w189, "正则表达式"="PlateSizeSKUforUIProvision</Name><Value>") -> ("匹配之后"=w192:string)  [unwired: 4 in, 4 out]
        n56 = xnode "匹配正则表达式"("输入字符串"=w189, "正则表达式"="PlateSizeforUIProvision</Name><Value>") -> ("匹配之后"=w193:string)  [unwired: 4 in, 4 out]
        n57 = xnode "匹配正则表达式"("输入字符串"=w189, "正则表达式"="<Name>DDMMotorSN_X692</Name><Value>") -> ("匹配之后"=w207:string)  [unwired: 4 in, 4 out]
        n58 = xnode "匹配正则表达式"("输入字符串"=w201, "正则表达式"="</Value>") -> ("匹配之前"=w198:string)  [unwired: 4 in, 4 out]
        n59 = xnode "匹配正则表达式"("输入字符串"=w193, "正则表达式"="</Value>") -> ("匹配之前"=w168:string)  [unwired: 4 in, 4 out]
        n60 = xnode "匹配正则表达式"("输入字符串"=w192, "正则表达式"="</Value>") -> ("匹配之前"=w176:string)  [unwired: 4 in, 4 out]
        n61 = xnode "匹配正则表达式"("输入字符串"=w207, "正则表达式"="</Value>") -> ("匹配之前"=w206:string)  [unwired: 4 in, 4 out]
        n62 = Empty String/Path?(string/path=w168) -> (empty?=w188:bool)
        n63 = Empty String/Path?(string/path=w176) -> (empty?=w187:bool)
        n64 = Concatenate Strings("'", w206) -> (w205:string)
        n65 = call "Read_Sku.vi"("SKU"=w176) -> ("Recipe"=w175:string)  [unwired: 10 in]
        n66 = Empty String/Path?(string/path=w175) -> (empty?=w174:bool)
        n67 = property class="CmbBox"(reference=w165, "Value"=w175) -> ()  [unwired: 1 in, 2 out]
        n68 = call "1-BasePath.vi"("Step"=enum16{"Initial", "Write", "Read"}."Read") -> ("Path Out"=w182:path)  [unwired: 9 in, 1 out]
        n69 = call "ReadConfigandSetting.vi"("Recipe"=w175, "Path Out"=w182) -> ("错误输出"=w173:errorcluster, "TableData"=w185:string[][])  [unwired: 7 in, 1 out]
        n70 = Search and Replace String(input string=w168, search string="mm" ("替换字符串(\"\")")) -> (result string=w171:string)  [unwired: 6 in, 3 out]
        n71 = Build Path(base path=w182, name or relative path="data\\Recipe.ini") -> ()  [unwired: 1 out]
        n72 = call "Index_Config.vi"("Action"="MAX_POWER_MODE_Orifice_size") -> ("data"=w170:string)  [unwired: 10 in]
        n73 = Not Equal?(x=w170, y=w171) -> (x != y?=w167:bool)
        n74 = Compound Arithmetic op=OR ("复合运算")(w167, w173, w174, w188, w187) -> (w186:bool)
        n75 = case shown="真" w219 {
          tunnel: w218 -> [w1144 w1145]
          tunnel: ["Wait_Scan_ProductID" ("Value") w1149] -> _
          tunnel: w197 -> [w1141 w1148]
          tunnel: w196 -> [w1140 w1147]
          tunnel: w186 -> [_ w1146]
          frame False {
            n76 = property class="Str"(reference=w1144, "Value"="" ("值")) -> ()  [unwired: 1 in, 2 out]
            n77 = property class="Str"(reference=w1141, "Value"=w1140, "Blinking"=FALSE ("闪烁")) -> ()  [unwired: 1 in, 2 out]
          }
          frame True {
            n78 = case shown="真" w1146 {
              tunnel: ["Check_Carrier_Sensor_Signal" "Wait_Scan_ProductID" ("Value")] -> w1149
              tunnel: w1148 -> [w1151 w1154]
              tunnel: w1147 -> [w1150 _]
              tunnel: w1145 -> [_ w1157]
              frame False {
                n79 = property class="Str"(reference=w1151, "Value"=w1150) -> ()  [unwired: 1 in, 2 out]
              }
              frame True {
                n80 = property class="Str"(reference=w1157, "Value"="" ("值")) -> ()  [unwired: 1 in, 2 out]
                n81 = property class="字符串"(reference=w1154, "Value"="0; SKU or PlateSize Data Error" ("字符串"), "Blinking"=FALSE ("闪烁")) -> ()  [unwired: 1 in, 2 out]
              }
            }
          }
        }
        n82 = Delete From Array(array=w185, length=1 ("长度"), index (row)=0 ("索引 (行)")) -> (deleted portion=w183:string[][], array with subset deleted=w184:string[][])  [unwired: 1 in]
        n83 = call "Select_UUT_Table.vi"("all Title"=w183, "all Table"=w184) -> ("Table"=w177:string[][])  [unwired: 8 in, 1 out]
        n84 = Bundle By Name(cluster=w211, "MES DDM SN"=w205, "Retest"=w198, "Plate_Diameter"=w168, "SKU"=w176, "Table"=w177) -> (w210:T2)
        n85 = call "LogStatus.vi"("error in (no error)"=w225, "last message"=w221, "message"=w220) -> ("error  out"=w224:errorcluster)  [unwired: 8 in]
      }
      frame "Check_UUT_Sensor_Signal" {
        (unwired) "Wait_Start_signal"
        n86 = call "IO.vi"("IO Name"=string[] ["Photoelectric Presence Sensor"], "IO?"=enum16{"DI", "DO"}."DI") -> ("DI"=w1163:bool[])  [unwired: 7 in, 2 out]
        n87 = And Array Elements(Boolean array=w1163) -> (logical AND=w1162:bool)
        n88 = Select(t="Wait_Start_signal", s=w1162, f="Check_UUT_Sensor_Signal") -> (s? t:f=w1159:string)
        n89 = call "LogStatus.vi"("error in (no error)"=w1171, "last message"=w1164, "message"=w1165) -> ("error  out"=w1170:errorcluster)  [unwired: 8 in]
      }
      frame "Wait_Start_signal" {
        n90 = Unbundle By Name(w1176) -> ("Station ID"=w1177:string)
        "Station ID" <- w1177
        n91 = Unbundle By Name(w1180) -> ("Device state"=w1179:refnum<vi>)
        n92 = call "IO.vi"("IO Name"=string[] ["Start"], "IO?"=enum16{"DI", "DO"}."DI") -> ("DI"=w1181:bool[])  [unwired: 7 in, 2 out]
        n93 = And Array Elements(Boolean array=w1181) -> (logical AND=w1173:bool)
        n94 = case shown="真" w1173 {
          tunnel: w1179 -> [_ w1195]
          tunnel: w1176 -> [w1190 w1194]
          tunnel: [w1190 w1193] -> w1174
          tunnel: ["Wait_Start_signal" w1191] -> w1178
          tunnel: w1177 -> [_ _]
          frame False {
          }
          frame True {
            n95 = call "Cheak File.vi"() -> ("true"=w1192:bool)  [unwired: 11 in]
            n96 = case shown="假" w1192 {
              tunnel: w1195 -> [w1202 _]
              tunnel: w1194 -> [w1201 w1205]
              tunnel: [w1199 w1205] -> w1193
              tunnel: ["5.2.1Attachment_RFID_Detection_Test" ("Name") "Wait_Start_signal"] -> w1191
              frame False {
                n97 = Get Date/Time In Seconds() -> (seconds since 1Jan1904=w1200:timestamp)
                n98 = Bundle By Name(cluster=w1201, "Start Time"=w1200) -> (w1199:T2)
                n99 = call "Start.vi"("Start In"=TRUE, "Step"=enum16{"Initial", "Write", "Read"}."Write") -> ()  [unwired: 8 in, 2 out]
                n100 = call "StatusLamp.vi"("State"="Testing", "Boolean输入"=w1202) -> ()  [unwired: 9 in, 1 out]
              }
              frame True {
              }
            }
          }
        }
        n101 = call "LogStatus.vi"("error in (no error)"=w1187, "last message"=w1182, "message"=w1183) -> ("error  out"=w1186:errorcluster)  [unwired: 8 in]
      }
      frame "5.2.1Attachment_RFID_Detection_Test" {
        n102 = call "LogStatus.vi"("error in (no error)"=w1220, "last message"=w1219, "message"=w1214) -> ("error  out"=w1213:errorcluster)  [unwired: 8 in]
        n103 = call "1.0.0_Initialisation.vi"("Data in"=w1208, "error in (no error)"=w1213, "AllControls In"=w1210, 10:w1206, "Message Queue out"=w1218) -> ("error out"=w1216:errorcluster, "Flow"=w1207:string, "Data"=w1215:T3, "Message Queue Out"=w1217:T5, "Data out"=w1209:T2)  [unwired: 2 in]
        n104 = Equal?(x="Error", y=w1207) -> (x = y?=w1211:bool)
        n105 = case shown="真" w1211 {
          frame False {
          }
          frame True {
            n106 = call "6-AlarmStatus.vi"("AlarmValue"=TRUE, "AlarmIndex"=AlarmIndex."Test Error", "Step"=enum16{"Initial", "Write", "Read"}."Write") -> ()  [unwired: 7 in, 2 out]
          }
        }
      }
      frame "Disconnect_UUT" {
        n107 = Unbundle By Name(w1228) -> ("OK/NG"=w1225:bool, "daemon reference"=w1231:refnum<k5>)
        n108 = case shown="假" w1225 {
          frame False {
            n109 = call "IO.vi"("DO DATA"=bool[] [FALSE, TRUE, FALSE], "IO Name"=string[] ["Green", "Red", "Yellow"], "IO?"=enum16{"DI", "DO"}."DO") -> ()  [unwired: 6 in, 3 out]
          }
          frame True {
            n110 = call "Start.vi"("Start In"=FALSE, "Step"=enum16{"Initial", "Write", "Read"}."Write") -> ()  [unwired: 8 in, 2 out]
          }
        }
        n111 = call "disconnect.vi"("daemon reference in"=w1231) -> ("error out"=w1227:errorcluster, "response"=w1226:string, "daemon reference out"=w1232:refnum<k5>)  [unwired: 7 in, 1 out]
        n112 = call <vilib>:"Clear Errors.vi"("error in (no error)"=w1227) -> ()  [unwired: 5 in, 2 out]
        n113 = case shown="假" w1225 {
          tunnel: w1232 -> [w1244 w1249]
          tunnel: w1228 -> [w1245 w1248]
          tunnel: [w1246 w1247] -> w1230
          tunnel: w1226 -> [_ _]
          frame False {
            n114 = Bundle By Name(cluster=w1245, "daemon reference"=w1244) -> (w1246:T2)
          }
          frame True {
            n115 = Bundle By Name(cluster=w1248, "daemon reference"=w1249) -> (w1247:T2)
          }
        }
        n116 = call "LogStatus.vi"("error in (no error)"=w1237, "last message"=w1234, "message"=w1235) -> ("error  out"=w1236:errorcluster)  [unwired: 8 in]
        n117 = Wait (ms)(milliseconds to wait=u32 20) -> ()  [unwired: 1 out]
      }
      frame "UI_Display_and_Save_Test_Data" {
        w1253 = "Wait_Scan_ProductID" ("Name")
        n118 = Unbundle By Name(w1259) -> ("Start Time"=w1282:timestamp, "Count"=w1281:T7, "OK/NG"=w1252:bool)
        n119 = Unbundle By Name(w1280) -> ("ProductID"=w1270:refnum<vi>, "MES bool"=w1272:refnum<vi>, "Device state"=w1273:refnum<vi>, "TestInfo"=w1277:refnum<vi>, "Current CT"=w1279:refnum<vi>)
        n120 = Get Date/Time In Seconds() -> (seconds since 1Jan1904=w1287:timestamp)
        n121 = Subtract(x=w1287, y=w1282) -> (x-y=w1274:dbl)
        n122 = property class="Str"(reference=w1270, "Value"="" ("值")) -> ()  [unwired: 1 in, 2 out]
        n123 = property class="DigNum (严格)"(reference=w1279, "Value"=w1274) -> ()  [unwired: 1 in, 2 out]
        n124 = Unbundle By Name(w1281) -> ("Total"=w1286:i32, "OK"=w1265:i32, "NG"=w1266:i32)
        n125 = Increment(x=w1286) -> (x+1=w1284:i32)
        n126 = Increment(x=w1265) -> (x+1=w1268:i32)
        n127 = Increment(x=w1266) -> (x+1=w1267:i32)
        n128 = case shown="真" FALSE {
          tunnel: w1273 -> [_ w1299]
          tunnel: w1252 -> [_ w1295]
          frame False {
          }
          frame True {
            n129 = Select(t="Pass" ("State"), s=w1295, f="Fail" ("State")) -> (s? t:f=w1298:string)
            n130 = call "StatusLamp.vi"("State"=w1298, "Boolean输入"=w1299) -> ()  [unwired: 9 in, 1 out]
          }
        }
        n131 = Select(t=w1268, s=w1252, f=w1265) -> (s? t:f=w1264:i32)
        n132 = Select(t=w1266, s=w1252, f=w1267) -> (s? t:f=w1263:i32)
        n133 = Divide(x=w1264, y=w1284) -> (x/y=w1285:dbl)
        n134 = Multiply(x=w1285, y=100.0) -> (x*y=w1262:dbl)
        n135 = Bundle By Name(cluster=w1281, "Total"=w1284, "OK"=w1264, "NG"=w1263, "Yield"=w1262) -> (w1276:T7)
        n136 = property class="Clust (严格)"(reference=w1277, "Value"=w1276) -> ()  [unwired: 1 in, 2 out]
        n137 = Bundle By Name(cluster=w1259, "CT"=w1274, "Count"=w1276) -> (w1260:T2)
        n138 = Wait (ms)(milliseconds to wait=u32 2000) -> ()  [unwired: 1 out]
        n139 = Flatten To XML(anything=w1260) -> (xml string=w1278:string)
        n140 = call "HD_Config.vi"("Step"=enum16{"Initial", "Write", "Read"}."Read") -> ("HD Config out"=w1257:T4)  [unwired: 9 in, 1 out]
        n141 = case shown="假" w1252 {
          frame False {
          }
          frame True {
            n142 = call "Start.vi"("Start In"=FALSE, "Step"=enum16{"Initial", "Write", "Read"}."Write") -> ()  [unwired: 8 in, 2 out]
          }
        }
        n143 = call "AMC Send Local Message.vi"("Message Value"=w1278, "Message Name"="Save", "Message Queue in"=w1293) -> ()  [unwired: 7 in, 2 out]
        n144 = property class="Bool (严格)"(reference=w1272) -> ("Value"=w1271:bool)  [unwired: 1 in, 2 out]
        n145 = Unbundle By Name(w1257) -> ("GRR"=w1256:bool)
        n146 = Select(t="Upload_MES_System", s=w1271, f=w1253) -> (s? t:f=w1254:string)
        n147 = call "LogStatus.vi"("error in (no error)"=w1291, "last message"=w1288, "message"=w1289) -> ("error  out"=w1290:errorcluster)  [unwired: 8 in]
        n148 = Select(t="Wait_Scan_ProductID" ("Name"), s=w1256, f=w1254) -> ()  [unwired: 1 out]
      }
      frame "Upload_MES_System" {
        n149 = Unbundle By Name(w1305) -> ("MES"=w1304:bool)
        n150 = Unbundle By Name(w1302) -> ("SN"=w1309:string, "OK/NG"=w1317:bool)
        n151 = Format Date/Time String(time format string (%c)="%H%M%S" ("时间格式字符串(%c)")) -> (date/time string=w1310:string)  [unwired: 2 in]
        n152 = call "PathChoose.vi"(11:PathChoose."TestData") -> ("Path_Out"=w1313:path)  [unwired: 10 in]
        n153 = Concatenate Strings(w1309, "_" ("字符串"), w1310, ".csv" ("字符串")) -> (w1307:string)
        n154 = call "Data_Table.vi"("AllControls In"=w1303, "Data in"=w1302) -> ("Data out"=w1316:string[][])  [unwired: 9 in]
        n155 = Build Path(base path=w1313, name or relative path=w1307) -> (appended path=w1312:path)
        n156 = case shown="假" w1304 {
          tunnel: w1303 -> [w1332 _]
          tunnel: w1317 -> [w1328 _]
          tunnel: w1316 -> [w1327 _]
          tunnel: w1309 -> [w1326 _]
          frame False {
            n157 = call "Save Result.vi"("Data"=w1327, "布尔"=w1328, "ProductID"=w1326) -> ("结果字符串"=w1330:string)  [unwired: 5 in, 3 out]
            n158 = Unbundle By Name(w1332) -> ("MES"=w1331:refnum<vi>)
            n159 = Not Equal?(x=w1330, y="0") -> (x != y?=w1329:bool)
            n160 = property class="Str"(reference=w1331, "Value"=w1330, "Blinking"=w1329) -> ()  [unwired: 1 in, 2 out]
          }
          frame True {
          }
        }
        n161 = call-poly <vilib>:"Write Delimited Spreadsheet.vi"("file path (dialog if empty)"=w1312, "2D data"=w1316, "delimiter (\\t)"="," ("delimiter (\\t)")) -> ()  [unwired: 11 in, 2 out]
        n162 = call "LogStatus.vi"("error in (no error)"=w1323, "last message"=w1320, "message"=w1319) -> ("error  out"=w1322:errorcluster)  [unwired: 8 in]
      }
      frame "Error" {
        n163 = Unbundle By Name(w1336) -> ("daemon reference"=w1345:refnum<k5>)
        n164 = Unbundle By Name(w1352) -> ("Device state"=w1338:refnum<vi>, "ProductID"=w1351:refnum<vi>)
        n165 = property class="Str"(reference=w1351) -> ("Value"=w1350:string)  [unwired: 1 in, 2 out]
        n166 = Not A Number/Path/Refnum?(number/path/refnum=w1345) -> (NaN/Path/Refnum?=w1344:bool)
        n167 = Empty String/Path?(string/path=w1350) -> (empty?=w1349:bool)
        n168 = Select(t="Off_Power_Supply_Output", s=w1344, f="Disconnect_UUT") -> (s? t:f=w1342:string)
        n169 = call "6-AlarmStatus.vi"("Step"=enum16{"Initial", "Write", "Read"}."Read") -> ("AlarmValue Out"=w1347:bool[])  [unwired: 9 in, 1 out]
        n170 = call "IO.vi"("IO Name"=string[] ["Reset"], "IO?"=enum16{"DI", "DO"}."DI") -> ("DI"=w1358:bool[])  [unwired: 7 in, 2 out]
        n171 = Or Array Elements(Boolean array=w1347) -> (logical OR=w1340:bool)
        n172 = And Array Elements(Boolean array=w1358) -> (logical AND=w1339:bool)
        n173 = Not(x=w1340) -> (.not. x?=w1337:bool)
        n174 = Select(t="Initialize_UI" ("Name"), s=w1349, f=w1342) -> (s? t:f=w1355:string)
        n175 = And(x=w1337, y=w1339) -> ()  [unwired: 1 out]
        n176 = call "IO.vi"("DO DATA"=bool[] [FALSE, TRUE, FALSE], "IO Name"=string[] ["Green", "Red", "Yellow"], "IO?"=enum16{"DI", "DO"}."DO") -> ()  [unwired: 6 in, 3 out]
        n177 = Select(t=w1355, s=w1337, f="Error" ("Name")) -> (s? t:f=w1353:string)
        n178 = case shown="真" w1337 {
          tunnel: w1338 -> [_ w1365]
          frame False {
          }
          frame True {
            n179 = call "StatusLamp.vi"("State"="Testing", "Boolean输入"=w1365) -> ()  [unwired: 9 in, 1 out]
          }
        }
        n180 = call "LogStatus.vi"("error in (no error)"=w1363, "last message"=w1360, "message"=w1361) -> ("error  out"=w1362:errorcluster)  [unwired: 8 in]
      }
      frame "Exit_AutoRun" {
        n181 = TCP Close Connection(connection ID=w1369, error in (no error)=w1368) -> ()  [unwired: 1 in, 2 out]
        n182 = case shown="真" FALSE {
          frame False {
          }
          frame True {
            n183 = call "IO.vi"("DO DATA"=bool[] [FALSE, FALSE, TRUE], "IO Name"=string[] ["Green", "Red", "Yellow"], "IO?"=enum16{"DI", "DO"}."DO") -> ("error out"=w1377:errorcluster)  [unwired: 6 in, 2 out]
            n184 = call <vilib>:"Clear Errors.vi"("error in (no error)"=w1377) -> ()  [unwired: 5 in, 2 out]
          }
        }
        n185 = call "LogStatus.vi"("error in (no error)"=w1371, "message"=w1374) -> ("error  out"=w1373:errorcluster)  [unwired: 9 in]
      }
    }
    n186 = call "Exit.vi"("Step"=enum16{"Initial", "Write", "Read"}."Read" ("step")) -> ("Exit Out"=w46:bool)  [unwired: 9 in, 1 out]
    n187 = Compound Arithmetic op=OR(w38, w46) -> (w47:bool)
    n188 = call "AMC Run Step.vi"("Message Queue In"=w41, "Message Name"=w35, "Message Value"=w34, "error in (no error)"=w36, "Mli/Sig"=FALSE) -> ("Message Queue Out"=w48:T5, "error out"=w49:errorcluster)  [unwired: 13 in]
  }
  n189 = while {
    tunnel: w19 -> [w1387]
    tunnel: "AllControls In" -> [w1382]
    tunnel: [w1381] -> w4
    stop <- w1388 stop-if-true
    n190 = call "AMC Read Next Message.vi"("timeout (1ms)"=100, "Message Queue in"=w1387) -> ("Message Value"=w1383:string, "Message Name"=w1386:string, "Message Queue out"=w1381:T5)  [unwired: 2 in, 5 out]
    n191 = Wait (ms)(milliseconds to wait=u32 1) -> ()  [unwired: 1 out]
    n192 = case shown="\"Save\"" w1386 {
      tunnel: w1383 -> [_ _ w1396]
      tunnel: w1382 -> [_ _ w1395]
      frame "Null", Default {
      }
      frame "Wait" {
      }
      frame "Save" {
        n193 = Unflatten From XML(xml string=w1396, type=T2 {"SN"="", "Table"=[], "Count"={"Total"=0, "OK"=0, "NG"=0, "Yield"=0.0}, "Start Time"=timestamp(0 s since 1904-01-01), "daemon reference"=refnum, "CT"=0.0, "OK/NG"=FALSE, "Station ID"="", "MES DDM SN"="", "MES PCBA SN"="", "Retest"="", "Attachment RFID detection"={"UID"="", "tag content"=""}, "SKU"="", "Plate_Diameter"="", "Alarm"=""} ("Data in")) -> (value=w1393:T2)  [unwired: 1 in, 1 out]
        n194 = call "Data_Save.vi"("AllControls In"=w1395, "Data in"=w1393) -> ()  [unwired: 10 in]
      }
    }
    n195 = call "Exit.vi"("Step"=enum16{"Initial", "Write", "Read"}."Read" ("step")) -> ("Exit Out"=w1390:bool)  [unwired: 9 in, 1 out]
    n196 = call "Stop.vi"("Step"=enum16{"Initial", "Write", "Read"}."Read") -> ("Stop Out"=w1389:bool)  [unwired: 9 in, 1 out]
    n197 = Compound Arithmetic op=OR(w1390, w1389) -> (w1388:bool)
  }
  n198 = Release Queue(queue=w4) -> ()  [unwired: 2 in, 3 out]
  n199 = Unbundle By Name(w9) -> ("daemon reference"=w18:refnum<k5>)
  n200 = Release Queue(queue=w6, error in (no error)=w5) -> ()  [unwired: 1 in, 3 out]
  n201 = call "daemon disconnect.vi"("daemon reference in"=w18) -> ("error out"=w17:errorcluster)  [unwired: 10 in]
  n202 = call <vilib>:"Clear Errors.vi"("error in (no error)"=w17) -> ()  [unwired: 5 in, 2 out]
